vi "File Dialog Replace.vi"(4 "pattern label":string, 5 "button label":string, 6 "pattern (all files)":string, 7 "prompt":string, 8 "error in":errorcluster, 10 "default name":string, 11 "start path":path=path "") -> (0 "error out":errorcluster, 2 "Cancel":bool, 3 "selected path":path)   [LabVIEW 2015]
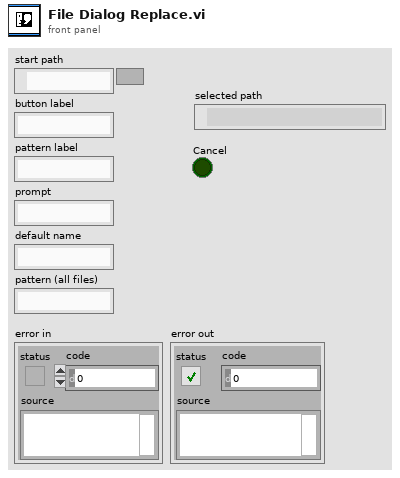
[diagram p1: front panel]
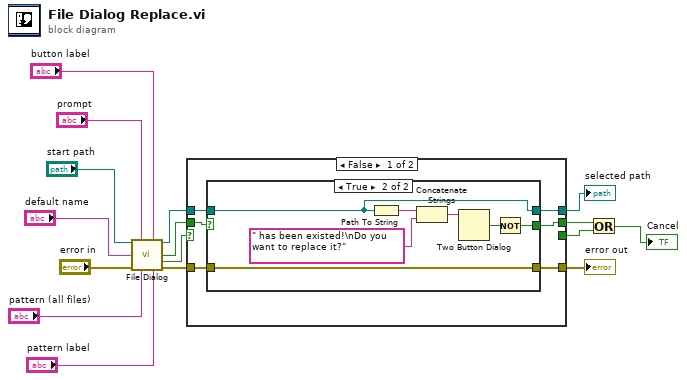
[diagram p0: block diagram]
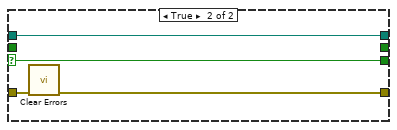
[diagram p3: hidden frame]
diagram:
  n1 = call "File Dialog"("start path"="start path", "prompt"="prompt", "button label"="button label", "default name"="default name", "error in"="error in", "pattern (all files)"="pattern (all files)", "pattern label"="pattern label") -> ("selected path"=w6:path, "exists"=w7:bool, "cancelled"=w9:bool, "error out"=w8:errorcluster)  [unwired: 5 in]
  n2 = case shown="False" w9 {
    selector: w9 -> [_ w32]
    tunnel: w8 -> [w20 w35]
    tunnel: [w19 w34] -> w5
    tunnel: w7 -> [w22 _]
    tunnel: w6 -> [w21 w33]
    tunnel: [w18 w33] -> w4
    tunnel: [_ w32] -> w2
    tunnel: [w17 _] -> w3
    frame False {
      n3 = case shown="True" w22 {
        tunnel: w21 -> [w23 w27]
        tunnel: w20 -> [w24 w28]
        tunnel: [w24 w28] -> w19
        tunnel: [w23 w27] -> w18
        tunnel: [_ w25] -> w17
        frame False {
        }
        frame True {
          n4 = Path To String(path=w27) -> (string=w31:string)
          n5 = Concatenate Strings(w31, " has been existed!\nDo you want to replace it?" ("string")) -> (w29:string)
          n6 = Two Button Dialog(message=w29) -> (T button?=w26:bool)  [unwired: 2 in]
          n7 = Not(x=w26) -> (.not. x?=w25:bool)
        }
      }
    }
    frame True {
      n8 = call <vilib>:"Clear Errors.vi"("error in (no error)"=w35) -> ("error out"=w34:errorcluster)  [unwired: 5 in, 1 out]
    }
  }
  "error out" <- w5
  "selected path" <- w4
  n9 = Or(x=w3, y=w2) -> (x .or. y?=→"Cancel":bool)
